vi "MakeOdorConcStrings.vi"(7 "Base Dilution":dbl=0.1, 8 "Concentration":u16[](array[ring])=[0, 1, 1, 1, 0, 0, 0, 1, 0, 0, 0, 0, 0] items=["10^-5", "10^-6", "Add new..."], 9 "Odor":u16[](array[ring])=[0, 1, 3, 2, 1, 0, 0, 0, 0, 0, 0, 0, 0] items=["1-pentanol", "3-pentanol", "3-octanol", "2,5-dimethylthiazole", "Add new..."], 10 "Concentration":refnum<vi>, 11 "Odor":refnum<vi>) -> (2 "Concentration Strings":string[](array[string])=["10^-5", "10^-6", "10^-6", "10^-6", "10^-5", "10^-5", "10^-5", "10^-6", "10^-5", "10^-5", "10^-5", "10^-5", "10^-5"], 3 "Odor Strings":string[](array[string])=["1-pentanol", "3-pentanol", "2,5-dimethylthiazole", "3-octanol", "3-pentanol", "1-pentanol", "1-pentanol", "1-pentanol", "1-pentanol", "1-pentanol", "1-pentanol", "1-pentanol", "1-pentanol"])   [LabVIEW 2016]
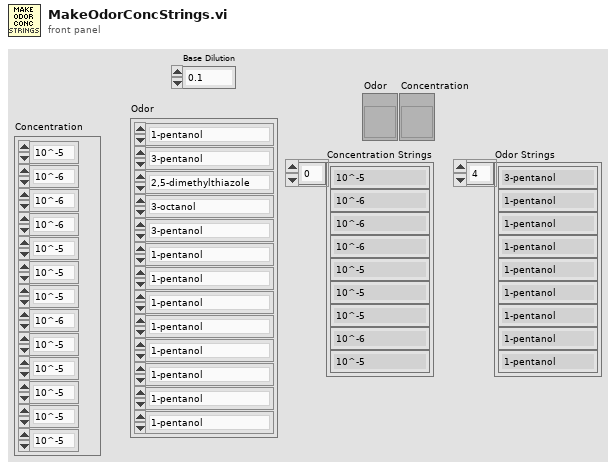
[diagram p1: front panel]
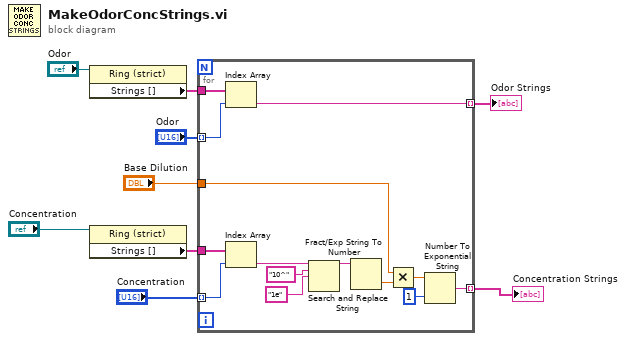
[diagram p0: block diagram]
diagram:
  n1 = property class="Ring (strict)"(reference="Odor") -> ("Strings []"=w8:string[])  [unwired: 1 in, 2 out]
  n2 = property class="Ring (strict)"(reference="Concentration") -> ("Strings []"=w9:string[])  [unwired: 1 in, 2 out]
  n3 = for {
    tunnel: "Odor" -> [w21] mode=indexing
    tunnel: w9 -> [w23]
    tunnel: w8 -> [w22]
    tunnel: [w20] -> w4 mode=indexing
    tunnel: [w11] -> w3 mode=indexing
    tunnel: "Concentration" -> [w19] mode=indexing
    tunnel: "Base Dilution" -> [w14]
    n4 = Index Array(array=w22, index=w21) -> (element=w20:string)
    n5 = Index Array(array=w23, index=w19) -> (element=w12:string)
    n6 = Search and Replace String(input string=w12, search string="10^", replace string="1e" ("replace string (\"\")")) -> (result string=w16:string)  [unwired: 5 in, 3 out]
    n7 = Fract/Exp String To Number(string=w16) -> (number=w15:dbl)  [unwired: 3 in, 1 out]
    n8 = Multiply(x=w14, y=w15) -> (x*y=w13:dbl)
    n9 = Number To Exponential String(number=w13, precision (6)=i16 1 ("width (-)")) -> (E-format string=w11:string)  [unwired: 2 in]
  }
  "Odor Strings" <- w4
  "Concentration Strings" <- w3
